vi "serialPARATIVA.vi"() -> ()   [LabVIEW 2018]
uses:
  <vilib>/Instr/_visa.llb/VISA Configure Serial Port (Instr).vi
panel:
  in  "stop":bool
  in  "baud rate (9600)":u32=9600
  in  "VISA resource name":refnum<visa-resource-name>
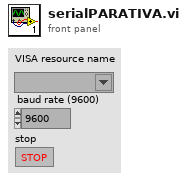
[diagram p1: front panel]
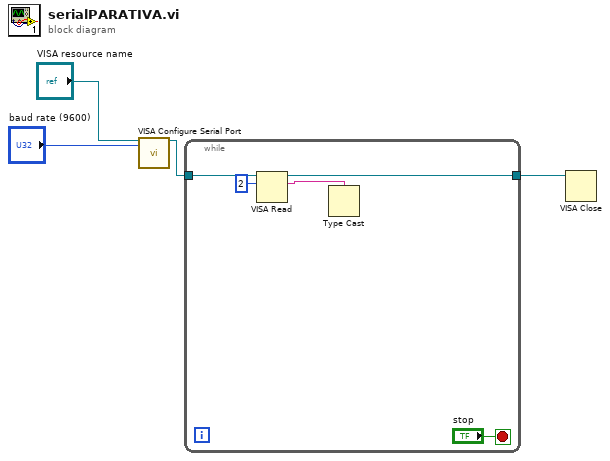
[diagram p0: block diagram]
diagram:
  n1 = call-poly "VISA Configure Serial Port"("VISA resource name"="VISA resource name", "baud rate (9600)"="baud rate (9600)") -> ("VISA resource name out"=w2:refnum<visa-resource-name>)  [unwired: 12 in, 1 out]
  n2 = while {
    tunnel: w2 -> [w8]
    tunnel: [w7] -> w1
    stop <- "stop" stop-if-true
    n3 = VISA Read(VISA resource name=w8, byte count=u32 2) -> (VISA resource name out=w7:refnum<visa-resource-name>, read buffer=w5:string)  [unwired: 1 in, 2 out]
    n4 = Type Cast(type=w5) -> ()  [unwired: 1 in, 1 out]
  }
  n5 = VISA Close(VISA resource name=w1) -> ()  [unwired: 1 in, 1 out]
